vi "Add Control to Events-Cluster.vi"(8 "error in (no error)":errorcluster, 10 "Control to Add":path, 11 "Events Type-Def Path":path) -> (0 "error out":errorcluster)   [LabVIEW 2018, in "Scripting.lvlib"]
uses:
  Scripting.lvlib
  <vilib>/Utility/traverseref.llb/TRef TravTarget.ctl
  <vilib>/Utility/miscctls.llb/LVPointTypeDef.ctl
  <vilib>/Utility/error.llb/Error Cluster From Error Code.vi
  <vilib>/ErrorRing/Error Ring.xnode
  <vilib>/Utility/traverseref.llb/VI Scripting - Traverse.lvlib
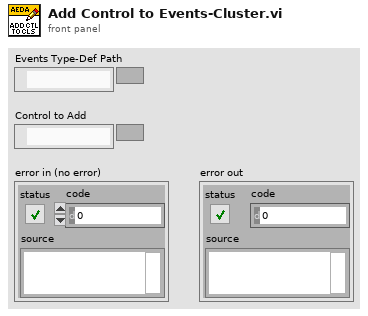
[diagram p1: front panel]
types:
  T1 = typedef "TRef TravTarget.ctl" = enum16{"FP", "BD", "Other"}
  T2 = typedef "LVPointTypeDef.ctl" = cluster{"Horizontal":i16, "Vertical":i16}
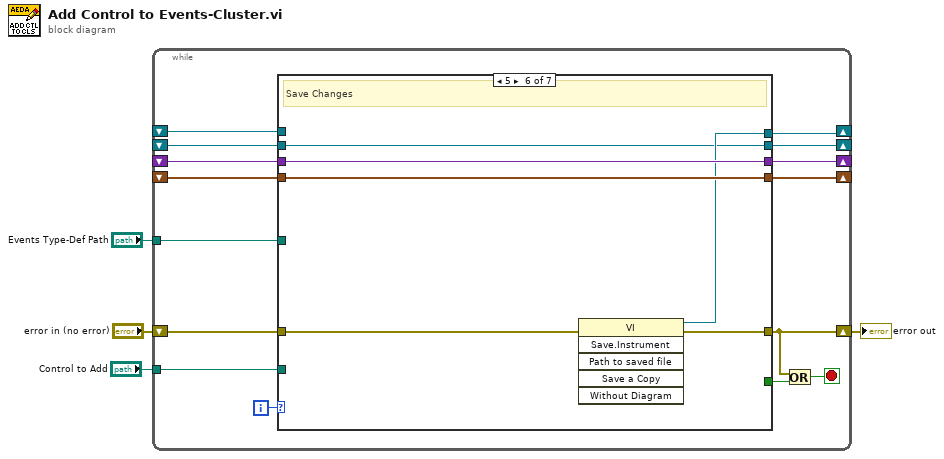
[diagram p0: block diagram]
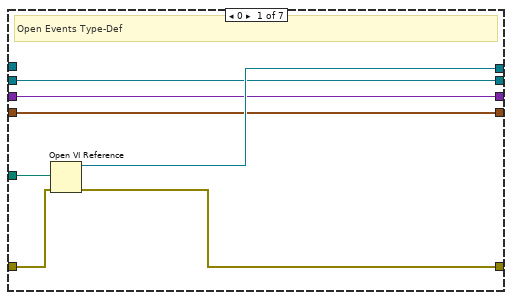
[diagram p2: hidden frame]
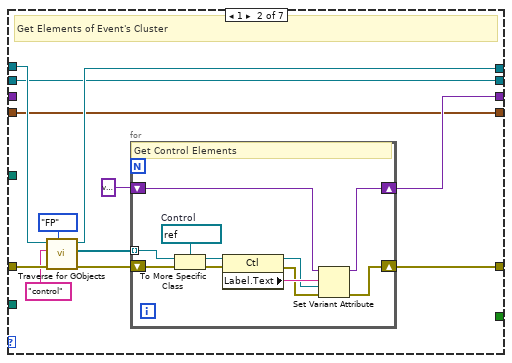
[diagram p3: hidden frame]
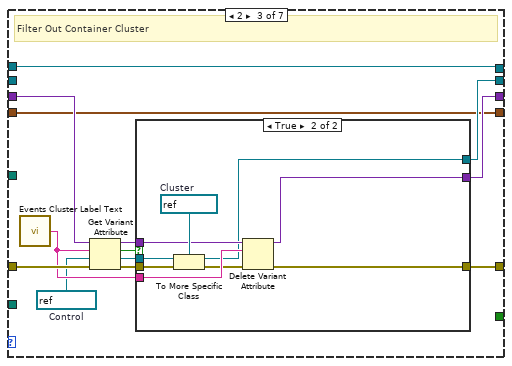
[diagram p4: hidden frame]
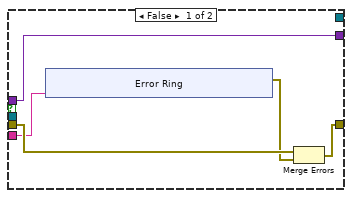
[diagram p5: hidden frame]
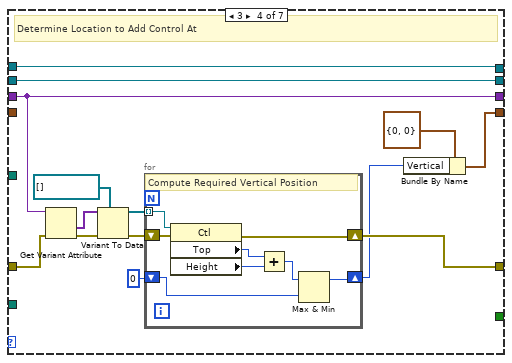
[diagram p6: hidden frame]
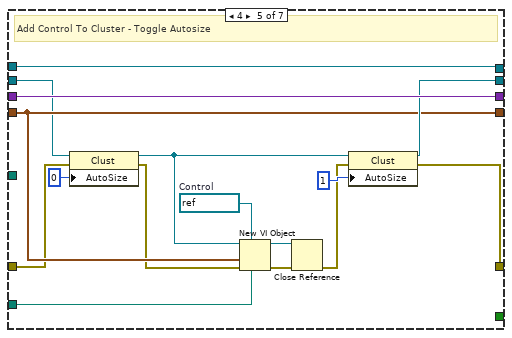
[diagram p7: hidden frame]
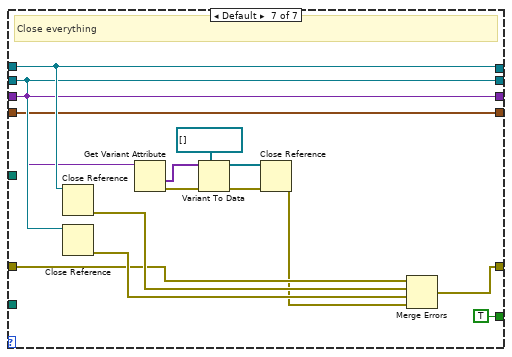
[diagram p8: hidden frame]
diagram:
  n1 = while {
    tunnel: "Events Type-Def Path" -> [w16]
    shift-right: [w15] -> _
    shift-left: _ -> [w14]
    shift-right: [w13] -> w4
    shift-left: "error in (no error)" -> [w12]
    shift-right: [w11] -> _
    shift-left: _ -> [w10]
    shift-right: [w9] -> _
    shift-left: _ -> [w8]
    shift-right: [w7] -> _
    shift-left: _ -> [w6]
    tunnel: "Control to Add" -> [w5]
    i -> [w19]
    stop <- w17 stop-if-true
    n2 = case shown="5" w19 {
      tunnel: [_ _ _ _ _ _ TRUE] -> w18
      tunnel: w16 -> [w26 _ _ _ _ _ _]
      tunnel: [w23 w34 w52 w88 w120 w125 w141] -> w15
      tunnel: w14 -> [_ w36 w52 w88 w120 _ w141]
      tunnel: [w24 w30 w55 w89 w112 w124 w136] -> w13
      tunnel: w12 -> [w25 w37 w59 w90 w110 w123 w137]
      tunnel: [w21 w29 w54 w91 w121 w127 w133] -> w11
      tunnel: w10 -> [w21 _ w60 w91 w121 w127 w133]
      tunnel: [w22 w28 w51 w87 w114 w122 w140] -> w9
      tunnel: w8 -> [w22 w28 _ w87 w108 w122 w140]
      tunnel: [w20 w27 w50 w86 w113 w126 w128] -> w7
      tunnel: w6 -> [w20 w27 w50 _ w113 w126 w128]
      tunnel: w5 -> [_ _ _ _ w119 _ _]
      frame 0 {
        # "Open Events Type-Def"
        n3 = Open VI Reference(vi path=w26, error in (no error)=w25) -> (vi reference=w23:refnum<vi>, error out=w24:errorcluster)  [unwired: 4 in]
      }
      frame 1 {
        # "Get Elements of Event's Cluster"
        n4 = call <vilib>:"Traverse for GObjects.vi"("Traverse Target"=TRef_TravTarget."FP", "error in (no error)"=w37, "Class Name"="control", "VI Refnum"=w36) -> ("error out"=w32:errorcluster, "References"=w31:refnum<vi>[], "dup VI Refnum"=w34:refnum<vi>)  [unwired: 4 in, 1 out]
        n5 = for {
          tunnel: w31 -> [w49] mode=indexing
          shift-right: [w41] -> w29
          shift-left: variant ("variant") -> [w42]
          shift-right: [w39] -> w30
          shift-left: w32 -> [w47]
          w48 = refnum<vi> refnum  # Control
          # "Get Control Elements"
          n6 = To More Specific Class(target class=w48, reference=w49, error in=w47) -> (specific class reference=w46:refnum<vi>, error out=w45:errorcluster)
          n7 = property class="Ctl"(reference=w46, error in=w45) -> (reference out=w43:refnum<vi>, error out=w40:errorcluster, "Label.Text"=w44:string)
          n8 = Set Variant Attribute(Variant=w42, name=w44, value=w43, error in=w40) -> (Variant out=w41:variant, error out=w39:errorcluster)  [unwired: 1 out]
        }
      }
      frame 2 {
        w53 = refnum<vi> refnum  # Control
        # "Filter Out Container Cluster"
        n9 = call "Events Cluster Label Text.vi"() -> ("Events Cluster Label Text"=w57:string)
        n10 = Get Variant Attribute(Variant=w60, name=w57, default value (empty Variant)=w53, error in=w59) -> (duplicate Variant=w62:variant, found=w58:bool, value=w56:refnum<vi>, error out=w61:errorcluster)
        n11 = case shown="True" w58 {
          tunnel: w62 -> [w63 w78]
          tunnel: w61 -> [w67 w81]
          tunnel: w57 -> [w65 w83]
          tunnel: w56 -> [_ w80]
          tunnel: [w64 w76] -> w55
          tunnel: [w63 w77] -> w54
          tunnel: [_ w75] -> w51
          frame False {
            n12 = xnode "Error Ring"("parameter 0"=w65) -> ("error out"=w66:errorcluster)
            n13 = Merge Errors(w67, w66) -> (w64:errorcluster)
          }
          frame True {
            w82 = refnum<vi> refnum  # Cluster
            n14 = To More Specific Class(target class=w82, reference=w80, error in=w81) -> (specific class reference=w75:refnum<vi>, error out=w79:errorcluster)
            n15 = Delete Variant Attribute(4:w79, 6:w83, 7:w78) -> (0:w76:errorcluster, 3:w77:variant)  [unwired: 1 out]
          }
        }
      }
      frame 3 {
        # "Determine Location to Add Control At"
        n16 = Get Variant Attribute(Variant=w91, error in=w90) -> (values=w94:variant[], error out=w95:errorcluster)  [unwired: 2 in, 2 out]
        n17 = Variant To Data(error in=w95, type=refnum<vi>[] [], Variant=w94) -> (data=w97:refnum<vi>[], error out=w96:errorcluster)
        n18 = for {
          shift-right: [w98] -> w89
          shift-left: w96 -> [w105]
          shift-right: [w101] -> w84
          shift-left: u32 0 -> [w100]
          tunnel: w97 -> [w99] mode=indexing
          # "Compute Required Vertical Position"
          n19 = property class="Ctl"(reference=w99, error in=w105) -> (error out=w98:errorcluster, "Top"=w104:i32, "Height"=w103:u32)  [unwired: 1 out]
          n20 = Add(x=w104, y=w103) -> (x+y=w102:u32)
          n21 = Max & Min(x=w102, y=w100) -> (max(x,y)=w101:u32)  [unwired: 1 out]
        }
        n22 = Bundle By Name(cluster=T2 {"Horizontal"=0, "Vertical"=0} ("location"), "Vertical"=w84) -> (w86:T2)
      }
      frame 4 {
        w111 = refnum<vi> refnum  # Control
        # "Add Control To Cluster - Toggle Autosize"
        n23 = property class="Clust"(reference=w108, error in=w110, "AutoSize"=u32 0 ("Auto Sizing")) -> (reference out=w107:refnum<vi>, error out=w109:errorcluster)
        n24 = New VI Object(vi object class=w111, owner refnum=w107, position/next to=w113, 6:w119, 8:w109) -> (object refnum=w116:refnum<vi>, 0:w117:errorcluster)  [unwired: 3 in]
        n25 = Close Reference(reference=w116, error in (no error)=w117) -> (error out=w115:errorcluster)
        n26 = property class="Clust"(reference=w107, error in=w115, "AutoSize"=u32 1 ("Auto Sizing")) -> (reference out=w114:refnum<vi>, error out=w112:errorcluster)
      }
      frame 5 {
        # "Save Changes"
        n27 = invoke class="VI" method="Save.Instrument"(error in=w123) -> (reference out=w125:refnum<vi>, error out=w124:errorcluster)  [unwired: 5 in, 4 out]
      }
      frame Default {
        # "Close everything"
        n28 = Close Reference(reference=w141) -> (error out=w139:errorcluster)  [unwired: 1 in]
        n29 = Close Reference(reference=w140) -> (error out=w138:errorcluster)  [unwired: 1 in]
        n30 = Get Variant Attribute(Variant=w133) -> (values=w134:variant[], error out=w135:errorcluster)  [unwired: 3 in, 2 out]
        n31 = Variant To Data(error in=w135, type=refnum<vi>[] [], Variant=w134) -> (data=w131:refnum<vi>[], error out=w130:errorcluster)
        n32 = Close Reference(reference=w131, error in (no error)=w130) -> (error out=w129:errorcluster)
        n33 = Merge Errors(w137, w139, w138, w129) -> (w136:errorcluster)
      }
    }
    n34 = Or(x=w13, y=w18) -> (x .or. y?=w17:bool)
  }
  "error out" <- w4
